vi "Bind Control Caption.vi"(4 "Ignore Past Updates? (F)":bool, 8 "error in (no error)":errorcluster, 9 "Datum Name (\"\"=Use Control Label)":string, 10 "Control Refnum":refnum<vi>, 11 "IViewable in":refnum<class "IViewable.lvclass">) -> (0 "error out":errorcluster, 3 "IViewable out":refnum<class "IViewable.lvclass">)   [LabVIEW 2015, in "IViewable.lvlib" / "IViewable.lvclass"]
doc: "<License>\nCopyright © 2017 Composed Systems, LLC | All rights reserved\nwww.composed.io\n\nAuthor: Ethan Stern <ethan.stern@composed.io>\n\nThis software is provided \"AS IS\" WITHOUT WARRANTIES, either express or implied, AND IS FOR EDUCATIONAL PURPOSES ONLY.\n</License>"
uses:
  IViewable.lvclass
  <vilib>/ActorFramework/Actor/Actor.lvclass/Actor.ctl
  <vilib>/ActorFramework/Message Enqueuer/Message Enqueuer.lvclass/Message Enqueuer.ctl
  SubscriptionPolicy/ValueChangeSubscription/ValueChangeSubscription.lvclass/ValueChangeSubscription.ctl
  IObserver/IObserver Messages/Subscribe Msg/Subscribe Msg.lvclass/Subscribe Msg.ctl
  <vilib>/ActorFramework/Message Enqueuer/Init from Existing Queue.vi
  <vilib>/ActorFramework/Message Enqueuer/Enqueue.vi
  <vilib>/ActorFramework/Message Priority Queue/Priority Enqueue.vi
  <vilib>/ActorFramework/Message Enqueuer/Message Enqueuer.lvclass
  SubscriptionPolicy/ValueChangeSubscription/ValueChangeSubscription.lvclass
  IObserver/IObserver Messages/Subscribe Msg/Subscribe Msg.lvclass
  IMediator/SubscriptionRequest/SubscriptionRequest.lvclass
  IObserver/IObserver/IObserver.lvclass
  <vilib>/ActorFramework/Actor/Actor.lvclass
  IMediator/ISubscriptionPolicy/ISubscriptionPolicy.lvclass
  Transport/ControlCaptionBinding/ControlCaptionBinding.lvclass
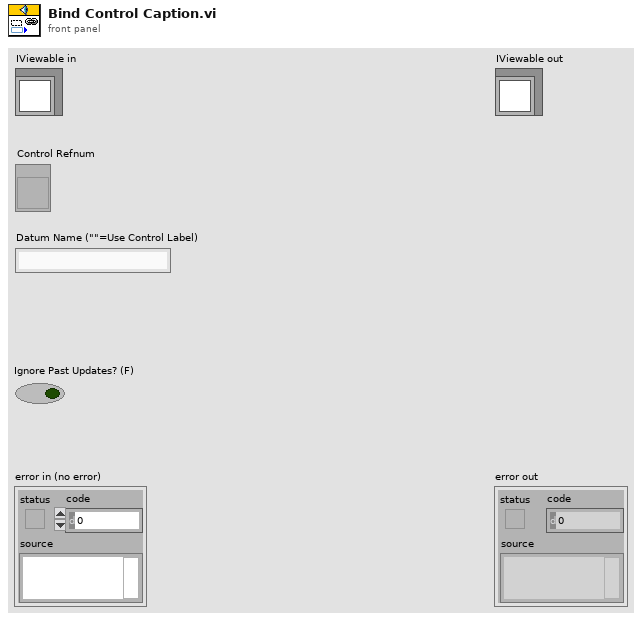
[diagram p1: front panel]
types:
  T1 = typedef "IMediator.lvlib/ISubscriptionPolicy.lvclass/ISubscriptionPolicy Reference.ctl" = refnum<data-value>
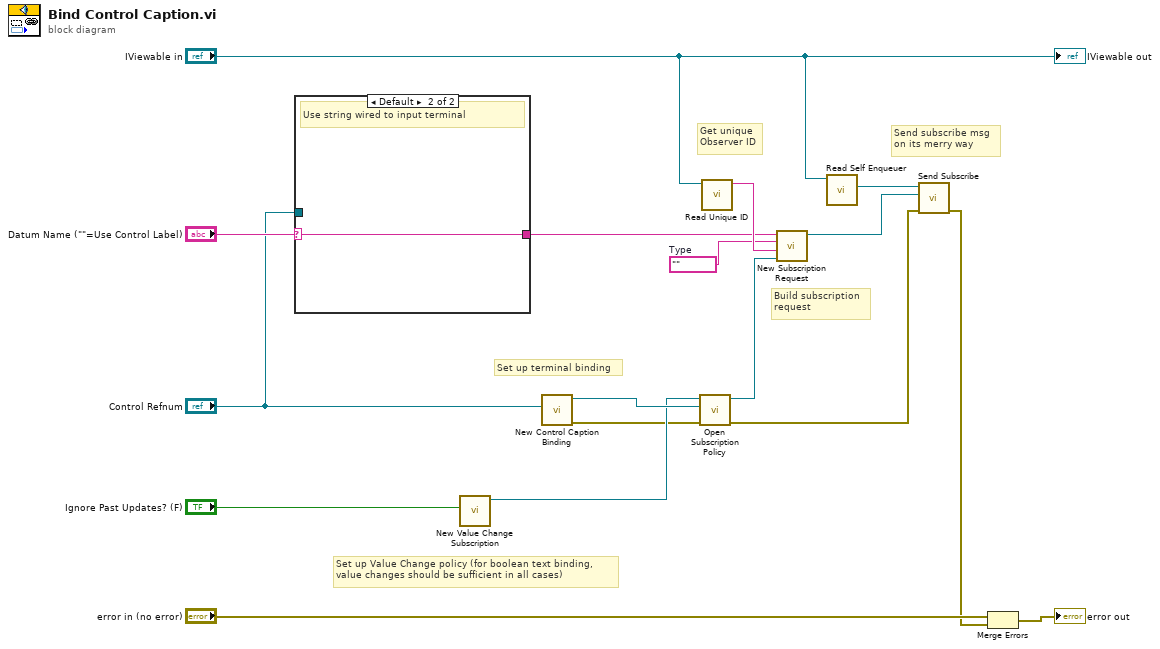
[diagram p0: block diagram]
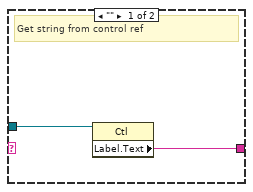
[diagram p2: hidden frame]
diagram:
  w3 = ""  # Type
  # "Set up Value Change policy (for boolean text binding,\nvalue changes should be sufficient in all cases)"
  # "Send subscribe msg\non its merry way"
  # "Build subscription\nrequest"
  # "Get unique\nObserver ID"
  # "Set up terminal binding"
  n1 = case shown="Default" "Datum Name (\"\"=Use Control Label)" {
    selector: "Datum Name (\"\"=Use Control Label)" -> [_ w20]
    tunnel: [w18 w20] -> w10
    tunnel: "Control Refnum" -> [w19 _]
    frame "" {
      # "Get string from control ref"
      n2 = property class="Ctl"(reference=w19) -> ("Label.Text"=w18:string)  [unwired: 1 in, 2 out]
    }
    frame Default {
      # "Use string wired to input terminal"
    }
  }
  n3 = call "New Value Change Subscription.vi"("Ignore Past Updates? (F)"="Ignore Past Updates? (F)") -> ("ValueChangeSubscription Out"=w4:refnum<class "ValueChangeSubscription.lvclass">)  [unwired: 10 in]
  n4 = call "New Control Caption Binding.vi"("Ctl Refnum"="Control Refnum") -> ("error out"=w2:errorcluster, "ControlCaptionBinding"=w7:refnum<class "ControlCaptionBinding.lvclass">)  [unwired: 9 in]
  n5 = call "Open Subscription Policy.vi"("error in (no error)"=w2, "Transport"=w7, "SubscriptionPolicy"=w4) -> ("error out"=w1:errorcluster, "Subscription Policy"=w8:T1)  [unwired: 7 in]
  n6 = call "Read Unique ID.vi"("IObserver In"="IViewable in") -> ("Unique ID"=w16:string)  [unwired: 10 in]
  n7 = call "New Subscription Request.vi"("Subscription Policy"=w8, "Subscriber ID"=w16, "Type"=w3, "Datum Name"=w10) -> ("SubscriptionRequest"=w6:refnum<class "SubscriptionRequest.lvclass">)  [unwired: 7 in]
  n8 = call <vilib>:"Read Self Enqueuer.vi"("Actor"="IViewable in") -> ("Self Enqueuer"=w14:refnum<class "Message Enqueuer.lvclass">)  [unwired: 10 in]
  n9 = call "Send Subscribe.vi"("error in (no error)"=w1, "SubscriptionRequest"=w6, "Message Enqueuer"=w14) -> ("error out"=w12:errorcluster)  [unwired: 7 in, 1 out]
  n10 = Merge Errors("error in (no error)", w12) -> (→"error out":errorcluster)
  "IViewable out" <- "IViewable in"
